vi "16.1 Locate the Edges.vi"() -> ()   [LabVIEW 2016]
uses:
  <vilib>/vision/Measure.llb/Edge Options.ctl
  <vilib>/vision/Measure.llb/Edge Polarity.ctl
  <vilib>/vision/NI_Vision_Development_Module.lvlib
panel:
  out "Image":T1(plugin-control)
  out "Coordinate System Out":T2 {"Measurement System"."Axis Reference" items=["Direct", "Indirect"]; "Measurement System"."Angle (deg)" format="%.2f"; "Measurement System"."Origin"."Y" format="%.2f"; "Measurement System"."Origin"."X" format="%.2f"; "Reference System"."Axis Reference" items=["Direct", "Indirect"]; "Reference System"."Angle (deg)" format="%.2f"; "Reference System"."Origin"."Y" format="%.2f"; "Reference System"."Origin"."X" format="%.2f"}
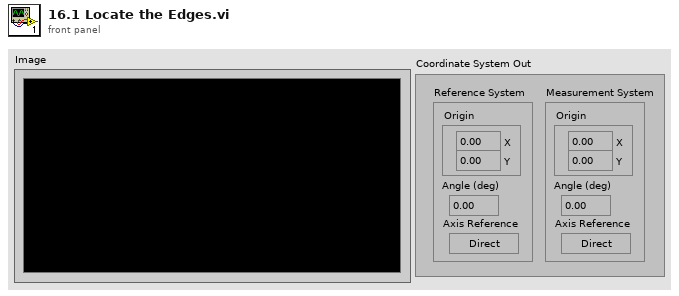
[diagram p1: front panel]
types:
  T1 = typedef "IMAQ Image.ctl" = refnum<image>
  T2 = typedef "IMAQ Coordinate System" = cluster{"Reference System":cluster{"Origin":cluster{"X":sgl, "Y":sgl}, "Angle (deg)":sgl, "Axis Reference":u32}, "Measurement System":cluster{"Origin":cluster{"X":sgl, "Y":sgl}, "Angle (deg)":sgl, "Axis Reference":u32}}
  T3 = typedef "IMAQ Rectangle" = cluster{"Left":i32, "Top":i32, "Right":i32, "Bottom":i32, "Rotation":dbl}
  T4 = typedef "Edge Options.ctl" = cluster{"Edge Polarity":T5, "Kernel Size":u32, "Width":u32, "Minimum Edge Strength":sgl, "Interpolation Type":enum32{"Zero Order", "Bilinear", "Quadratic", "Cubic", "Bilinear Fixed"}, "Data Processing Method":enum32{"Average", "Median"}}
  T5 = typedef "Edge Polarity.ctl" = u32
  T6 = cluster{"Direction":u16, "Primary Edge Options":T4, "Secondary Edge Options":T4, "Show Search Area":bool, "Show Search Lines":bool, "Show Edges Found":bool, "Show Result":bool, "Search Area Color":u32, "Search Lines Color":u32, "Edge Locations Color":u32, "Result Color":u32, "Overlay Group Name":string}
  T7 = typedef "ROI Descriptor" = cluster{"Global Rectangle":i32[], "Contours":cluster{"ID":enum32{"External", "Internal"}, "Type":u32, "Coordinates":i32[]}[]}
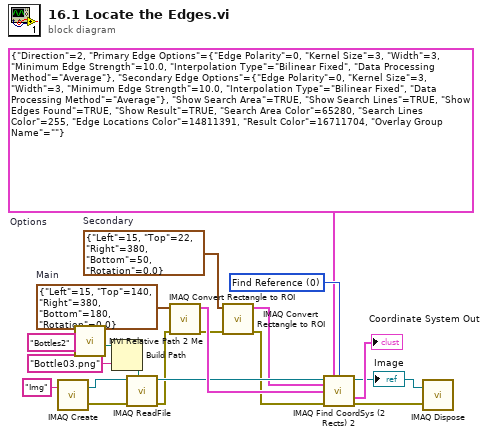
[diagram p0: block diagram]
diagram:
  w14 = T3 {"Left"=15, "Top"=140, "Right"=380, "Bottom"=180, "Rotation"=0.0}  # Main
  w15 = T3 {"Left"=15, "Top"=22, "Right"=380, "Bottom"=50, "Rotation"=0.0}  # Secondary
  w13 = T6 {"Direction"=2, "Primary Edge Options"={"Edge Polarity"=0, "Kernel Size"=3, "Width"=3, "Minimum Edge Strength"=10.0, "Interpolation Type"=enum."Bilinear Fixed", "Data Processing Method"=enum."Average"}, "Secondary Edge Options"={"Edge Polarity"=0, "Kernel Size"=3, "Width"=3, "Minimum Edge Strength"=10.0, "Interpolation Type"=enum."Bilinear Fixed", "Data Processing Method"=enum."Average"}, "Show Search Area"=TRUE, "Show Search Lines"=TRUE, "Show Edges Found"=TRUE, "Show Result"=TRUE, "Search Area Color"=65280, "Search Lines Color"=255, "Edge Locations Color"=14811391, "Result Color"=16711704, "Overlay Group Name"=""}  # Options
  w17 = u16 0 items=["Find Reference", "Update CoordSys"] ("Mode")
  n1 = call "IMAQ Create"("Image Name"="Img") -> ("Src"=w11:T1, "error out"=w12:errorcluster)  [unwired: 4 in]
  n2 = call "MVi Relative Path 2 Me.vi"("Relative Path"="Bottles2" ("name or relative path")) -> ("Appended Dir"=w20:path)  [unwired: 5 in, 1 out]
  n3 = Build Path(base path=w20, name or relative path="Bottle03.png") -> (appended path=w18:path)
  n4 = call "IMAQ ReadFile"("File Path"=w18, "error in (no error)"=w12, "Image"=w11) -> ("error out"=w4:errorcluster, "Image Out"=w8:T1)  [unwired: 4 in, 3 out]
  n5 = call "IMAQ Convert Rectangle to ROI"("error in (no error)"=w4, "Rectangle"=w14) -> ("error out"=w3:errorcluster, "ROI Descriptor"=w16:T7)  [unwired: 7 in]
  n6 = call "IMAQ Convert Rectangle to ROI"("error in (no error)"=w3, "Rectangle"=w15) -> ("error out"=w2:errorcluster, "ROI Descriptor"=w1:T7)  [unwired: 7 in]
  n7 = call "IMAQ Find CoordSys (2 Rects) 2"("Image"=w8, "Options"=w13, "Mode"=w17, "Primary ROI Descriptor"=w1, "Secondary ROI Descriptor"=w16, "error in (no error)"=w2) -> ("Image Out"=w5:T1, "Coordinate System Out"=→"Coordinate System Out":T2, "error out"=w7:errorcluster)  [unwired: 5 in, 2 out]
  "Image" <- w5
  n8 = call "IMAQ Dispose"("Image"=w5, "error in (no error)"=w7) -> ()  [unwired: 4 in, 1 out]
